vi "CONFOCAL MICROSCOPE-(NEW ALG).vi"() -> ()   [LabVIEW 2025]
uses:
  <vilib>/DAQmx/write.llb/DAQmx Write (Analog DBL 1Chan 1Samp).vi
  <vilib>/Analysis/1siggen.llb/Ramp Pattern by Samples.vi
  <vilib>/DAQmx/write.llb/DAQmx Write (Analog 1D Wfm NChan NSamp).vi
  <vilib>/DAQmx/read.llb/DAQmx Read (Counter 1D U32 1Chan NSamp).vi
  <vilib>/DAQmx/create/channels.llb/DAQmx Create Channel (AO-Voltage-Basic).vi
  <vilib>/DAQmx/configure/timing.llb/DAQmx Timing (Sample Clock).vi
  <vilib>/DAQmx/miscellaneous.llb/DAQmx Fill In Error Info.vi
  <vilib>/DAQmx/create/channels.llb/DAQmx Create Channel (CI-Count Edges).vi
  <vilib>/Analysis/NI_AALBase.lvlib
panel:
  in  "volts":dbl=1.0 format="%_2f"
  in  "pixels":dbl
  out "Intensity Graph":dbl[][](graph)
  out "appended array":dbl[][](array[numeric])
  out "transposed array":dbl[][](array[numeric])
  out "64bit integer":i64[](array[numeric])
  in  "Dwell time (s)":dbl
  out "Max Voltage (V)":dbl
  out "Min Voltage (V)":dbl
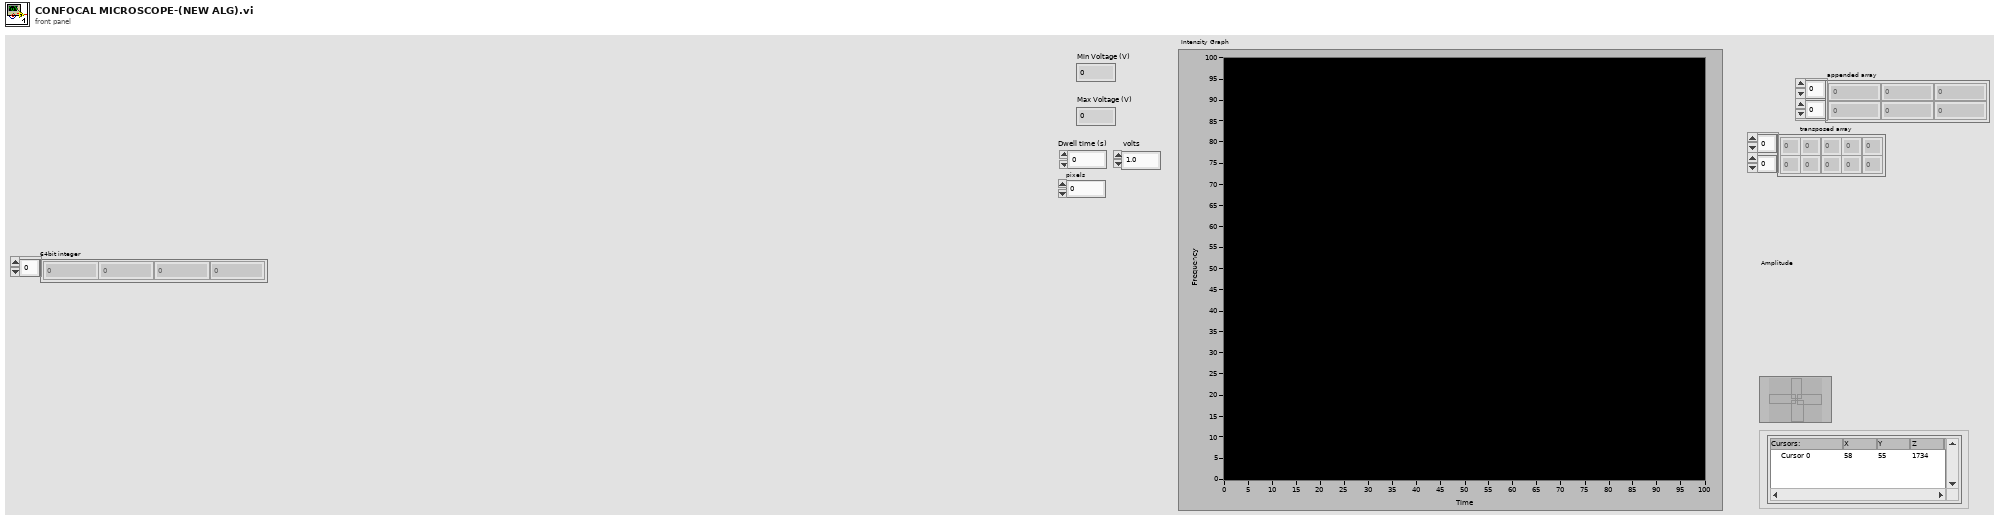
[diagram p1: front panel]
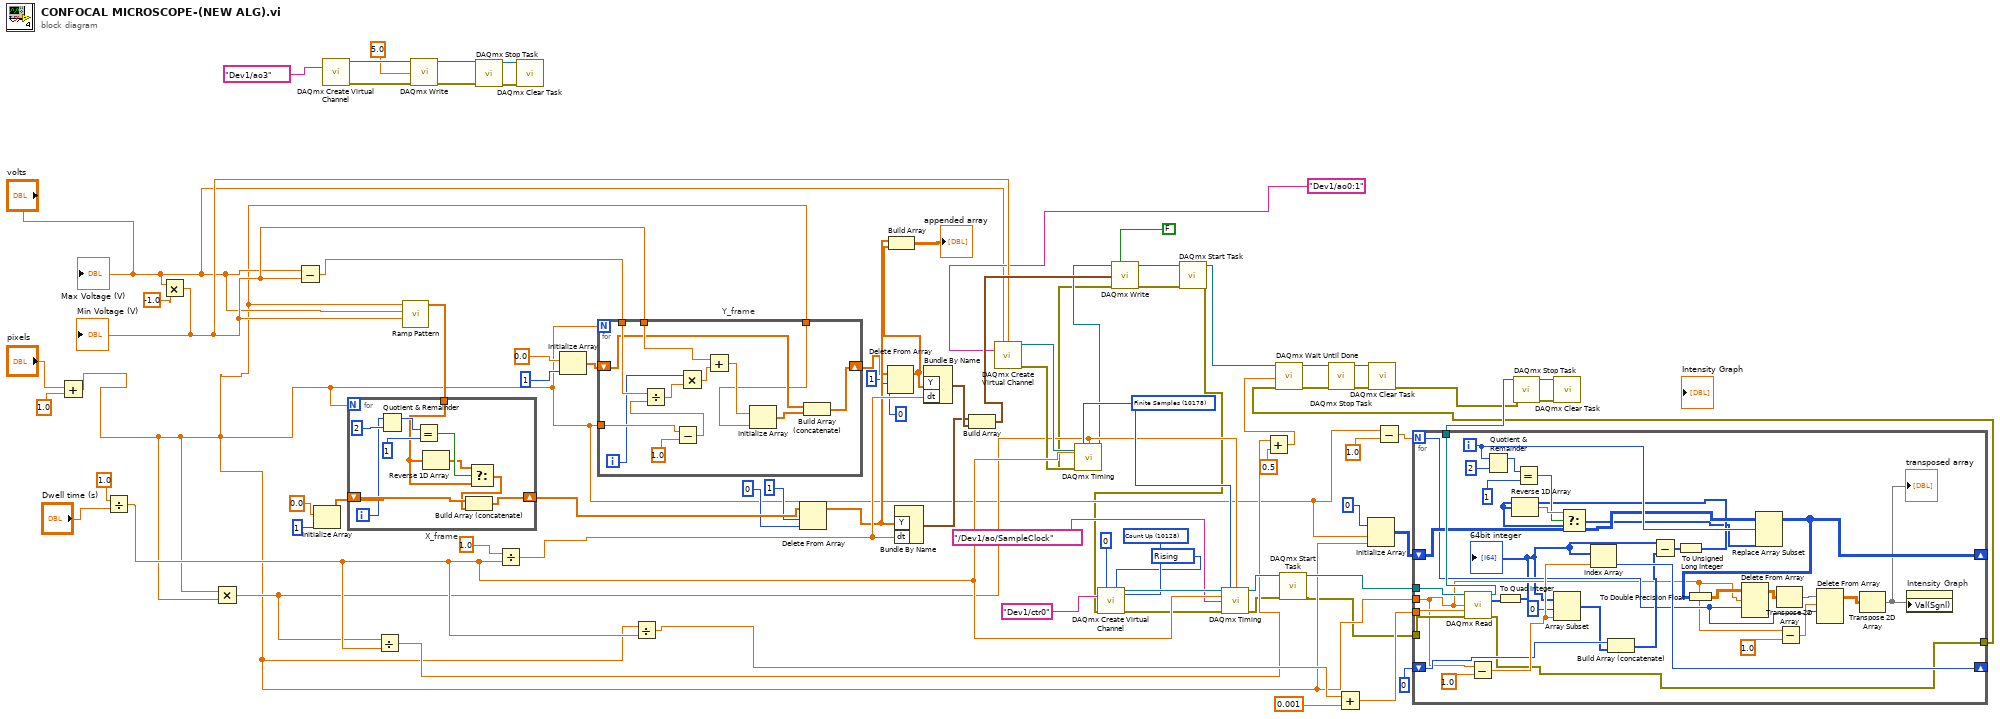
[diagram p0: block diagram]
diagram:
  w74 = 10178 items=["Finite Samples"=10178, "Continuous Samples"=10123, "Hardware Timed Single Point"=12522] ("Sample mode")
  w54 = 10280 items=["Rising"=10280, "Falling"=10171] ("edge")
  w55 = 10128 items=["Count Up"=10128, "Count Down"=10124, "Externally Controlled"=10326] ("count direction")
  n1 = Add(x="pixels", y=1.0) -> (x+y=w16:dbl)
  n2 = Divide(x=1.0, y="Dwell time (s)") -> (x/y=w39:dbl)
  n3 = Multiply(x="volts", y=-1.0) -> (x*y=w21:dbl)
  "Min Voltage (V)" <- w21
  n4 = Multiply(x=w16, y=w16) -> (x*y=w26:dbl)
  n5 = Subtract(x="volts", y=w21) -> (x-y=w15:dbl)
  n6 = Initialize Array(0.0 ("element"), 1 ("dimension size")) -> (w62:dbl[])
  n7 = call-poly <vilib>:"DAQmx Create Virtual Channel.vi"("physical channels"=tag "Dev1/ao3") -> ("task out"=w6:refnum<k21>, "error out"=w7:errorcluster)  [unwired: 13 in]
  n8 = Divide(x=w26, y=w39) -> (x/y=w25:dbl)
  n9 = call-poly <vilib>:"Ramp Pattern.vi"("start"=w21, "end"="volts", "samples"=w16) -> ("Ramp Pattern"=w78:dbl[])  [unwired: 7 in, 1 out]
  n10 = for "X_frame" {
    N: w16 -> [_]
    shift-right: [w91] -> w50
    shift-left: w62 -> [w92]
    tunnel: w78 -> [w85]
    i -> [w86]
    n11 = Quotient & Remainder(x=w86, y=2) -> (x-y*floor(x/y)=w89:i32)  [unwired: 1 out]
    n12 = Equal?(x=w89, y=1) -> (x = y?=w87:bool)
    n13 = Reverse 1D Array(array=w85) -> (reversed array=w84:dbl[])
    n14 = Select(t=w84, s=w87, f=w85) -> (s? t:f=w83:dbl[])
    n15 = Build Array (concatenate)(w92, w83) -> (w91:dbl[])
  }
  n16 = call-poly <vilib>:"DAQmx Write.vi"("task/channels in"=w6, "data"=5.0, "error in"=w7) -> ("task out"=w2:refnum<k21>, "error out"=w4:errorcluster)  [unwired: 10 in, 1 out]
  n17 = call <vilib>:"DAQmx Stop Task.vi"("task/channels in"=w2, "error in"=w4) -> ("task out"=w1:refnum<k21>, "error out"=w3:errorcluster)  [unwired: 12 in]
  n18 = Divide(x=1.0, y=w39) -> (x/y=w64:dbl)
  n19 = call <vilib>:"DAQmx Clear Task.vi"("task in"=w1, "error in"=w3) -> ()  [unwired: 13 in, 1 out]
  n20 = Initialize Array(0.0 ("element"), 1 ("dimension size")) -> (w63:dbl[])
  n21 = for "Y_frame" {
    N: w16 -> [_]
    tunnel: w16 -> [w105]
    tunnel: w15 -> [w103]
    tunnel: w21 -> [w98]
    tunnel: w16 -> [w93]
    shift-right: [w94] -> w46
    shift-left: w63 -> [w95]
    i -> [w100]
    n22 = Subtract(x=w105, y=1.0) -> (x-y=w102:dbl)
    n23 = Divide(x=w103, y=w102) -> (x/y=w101:dbl)
    n24 = Multiply(x=w100, y=w101) -> (x*y=w99:dbl)
    n25 = Add(x=w98, y=w99) -> (x+y=w97:dbl)
    n26 = Initialize Array(w97, w93) -> (w96:dbl[])
    n27 = Build Array (concatenate)(w95, w96) -> (w94:dbl[])
  }
  n28 = Divide(x=w16, y=w39) -> (x/y=w35:dbl)
  n29 = Delete From Array "Delete From Array"(array=w50, length=1, index=0) -> (array with subset deleted=w47:dbl[])  [unwired: 1 out]
  n30 = Delete From Array "Delete From Array"(array=w46, length=1, index=0) -> (array with subset deleted=w40:dbl[])  [unwired: 1 out]
  n31 = Build Array(w47, w40) -> (→"appended array":dbl[][])
  n32 = Bundle By Name("Y"=w47, "dt"=w64) -> (w65:waveform(dbl))  [unwired: 1 in]
  n33 = Bundle By Name("Y"=w40, "dt"=w64) -> (w66:waveform(dbl))  [unwired: 1 in]
  n34 = Build Array(w65, w66) -> (w68:waveform(dbl)[])
  n35 = call-poly <vilib>:"DAQmx Create Virtual Channel.vi"("maximum value"="volts", "minimum value"=w21, "physical channels"="Dev1/ao0:1" ("Galvo mirror path")) -> ("task out"=w67:refnum<k21>, "error out"=w33:errorcluster)  [unwired: 11 in]
  n36 = call-poly <vilib>:"DAQmx Timing.vi"("task/channels in"=w67, "sample mode"=w74, "samples per channel"=w26, "rate"=w39, "error in"=w33) -> ("task out"=w14:refnum<k21>, "error out"=w13:errorcluster)  [unwired: 9 in]
  n37 = call-poly <vilib>:"DAQmx Write.vi"("task/channels in"=w14, "auto start"=FALSE, "data"=w68, "error in"=w13) -> ("task out"=w69:refnum<k21>, "error out"=w12:errorcluster)  [unwired: 9 in, 1 out]
  n38 = call <vilib>:"DAQmx Start Task.vi"("task/channels in"=w69, "error in"=w12) -> ("task out"=w76:refnum<k21>, "error out"=w11:errorcluster)  [unwired: 12 in]
  n39 = call-poly <vilib>:"DAQmx Create Virtual Channel.vi"("initial count"=u32 0, "count direction"=w55, "edge"=w54, "counter"="Dev1/ctr0" ("Counter path"), "error in"=w11) -> ("task out"=w71:refnum<k21>, "error out"=w32:errorcluster)  [unwired: 9 in]
  n40 = call-poly <vilib>:"DAQmx Timing.vi"("task/channels in"=w71, "sample mode"=w74, "samples per channel"=w26, "rate"=w39, "source"=tag "/Dev1/ao/SampleClock", "error in"=w32) -> ("task out"=w72:refnum<k21>, "error out"=w10:errorcluster)  [unwired: 8 in]
  n41 = Add(x=w25, y=0.5) -> (x+y=w23:dbl)
  n42 = call <vilib>:"DAQmx Start Task.vi"("task/channels in"=w72, "error in"=w10) -> ("task out"=w73:refnum<k21>, "error out"=w9:errorcluster)  [unwired: 12 in]
  n43 = Add(x=w35, y=0.001) -> (x+y=w41:dbl)
  n44 = Initialize Array(u32 0 ("element"), w16, w16) -> (w75:u32[][])
  n45 = Subtract(x=w16, y=1.0) -> (x-y=w37:dbl)
  n46 = for {
    N: w37 -> [w112]
    tunnel: w16 -> [w108]
    tunnel: w41 -> [w139]
    tunnel: w73 -> [w138]
    shift-right: [w121] -> _
    shift-left: w75 -> [w124]
    tunnel: [w133] -> w34
    shift-right: [w130] -> _
    shift-left: u64 0 ("Numeric") -> [w128]
    tunnel: w9 -> [w119]
    tunnel: [w118] -> w27
    i -> [w125]
    n47 = call-poly <vilib>:"DAQmx Read.vi"("task/channels in"=w138, "number of samples per channel"=w108, "timeout"=w139, "error in"=w119) -> ("task out"=w133:refnum<k21>, "data"=w120:u32[], "error out"=w118:errorcluster)  [unwired: 9 in]
    n48 = Subtract(x=w108, y=1.0) -> (x-y=w129:dbl)
    n49 = Quotient & Remainder(x=w125, y=2) -> (x-y*floor(x/y)=w136:i32)  [unwired: 1 out]
    n50 = To Quad Integer(1:w120) -> (0:w106:i64[])
    "64bit integer" <- w106
    n51 = Equal?(x=w136, y=1) -> (x = y?=w132:bool)
    n52 = Array Subset "Array Subset"(array=w106, index=0, length=w129) -> (w107:i64[])
    n53 = Index Array "Index Array"(array=w106, index=w129) -> (element=w130:i64)
    n54 = Build Array (concatenate) "Build Array"(w128, w107) -> (w127:u64[])
    n55 = Subtract(x=w106, y=w127) -> (x-y=w126:u64[])
    n56 = To Unsigned Long Integer(number=w126) -> (unsigned 32bit integer=w123:u32[])
    n57 = Reverse 1D Array(array=w123) -> (reversed array=w134:u32[])
    n58 = Select(t=w134, s=w132, f=w123) -> (s? t:f=w122:u32[])
    n59 = Replace Array Subset "Replace Array Subset"(array=w124, new element=w122, index (row)=w125) -> (w121:u32[][])  [unwired: 1 in]
    n60 = To Double Precision Float(number=w121) -> (double precision float=w117:dbl[][])
    n61 = Delete From Array(array=w117, length=w108, index (row)=w112) -> (array with subset deleted=w116:dbl[][])  [unwired: 1 in, 1 out]
    n62 = Transpose 2D Array(2D array=w116) -> (transposed array=w115:dbl[][])
    n63 = Subtract(x=w108, y=1.0) -> (x-y=w113:dbl)
    n64 = Delete From Array(array=w115, length=w113, index (row)=w112) -> (array with subset deleted=w111:dbl[][])  [unwired: 1 in, 1 out]
    n65 = Transpose 2D Array(2D array=w111) -> (transposed array=w110:dbl[][])
    "transposed array" <- w110
    n66 = property on="Intensity Graph" class="IntGraph (strict)"("Val(Sgnl)"=w110) -> ()  [unwired: 2 in, 2 out]
  }
  n67 = call <vilib>:"DAQmx Wait Until Done.vi"("task/channels in"=w76, "timeout (sec)"=w23, "error in"=w27) -> ("task out"=w77:refnum<k21>, "error out"=w31:errorcluster)  [unwired: 11 in]
  n68 = call <vilib>:"DAQmx Stop Task.vi"("task/channels in"=w77, "error in"=w31) -> ("task out"=w70:refnum<k21>, "error out"=w30:errorcluster)  [unwired: 12 in]
  n69 = call <vilib>:"DAQmx Clear Task.vi"("task in"=w70, "error in"=w30) -> ("error out"=w29:errorcluster)  [unwired: 13 in]
  n70 = call <vilib>:"DAQmx Stop Task.vi"("task/channels in"=w34, "error in"=w29) -> ("task out"=w79:refnum<k21>, "error out"=w28:errorcluster)  [unwired: 12 in]
  n71 = call <vilib>:"DAQmx Clear Task.vi"("task in"=w79, "error in"=w28) -> ()  [unwired: 13 in, 1 out]
  "Max Voltage (V)" <- "volts"
